vi "Dequeue.vi"(8 "ErrorArray In":errorcluster[](array[cluster])) -> (0 "ErrorArray Out":errorcluster[](array[cluster]), 1 "Data":variant, 2 "Msg":string)   [LabVIEW 2014, in "Bus.lvlib" / "NISTBus.lvclass"]
uses:
  NISTBus.lvclass
  Framework/MsgQueue/TypeDef/MsgQueue.ctl
  <vilib>/Utility/error.llb/Error Cluster From Error Code.vi
  <vilib>/ErrorRing/Error Ring.xnode
  Framework/TestFramework.lvlib
  <userlib>/NIST/NISTErrorLib/NISTErrorLib.lvlib
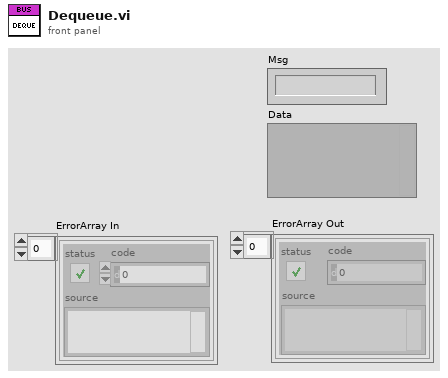
[diagram p1: front panel]
types:
  T1 = typedef "TestFramework.lvlib/MsgQueue.ctl" = cluster{"Msg":string, "Data":variant}
  T2 = typedef "TestFramework.lvlib/QueRef.ctl" = refnum<queue>
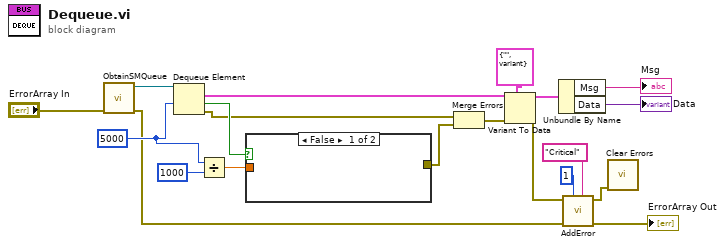
[diagram p0: block diagram]
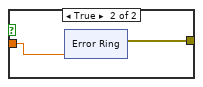
[diagram p2: hidden frame]
diagram:
  w17 = 5000 ("timeout in ms (-1)")
  n1 = call "ObtainSMQueue.vi"("ErrorArray In"="ErrorArray In") -> ("ErrorArray Out"=w4:errorcluster[], "QueRef"=w19:T2)  [unwired: 9 in]
  n2 = Dequeue Element(queue=w19, timeout in ms (-1)=w17) -> (element=w1:T1, timed out?=w16:bool, error out=w13:errorcluster)  [unwired: 1 in, 1 out]
  n3 = Divide(x=w17, y=1000) -> (x/y=w15:dbl)
  n4 = case shown="False" w16 {
    tunnel: w15 -> [_ w22]
    tunnel: [_ w21] -> w14
    frame False {
    }
    frame True {
      n5 = xnode "Error Ring"("parameter 0"=w22) -> ("error out"=w21:errorcluster)
    }
  }
  n6 = Merge Errors(w13, w14) -> (w12:errorcluster)
  n7 = Variant To Data(error in=w12, type=T1 {"Msg"="", "Data"=variant} ("MsgQueue"), Variant=w1) -> (data=w10:T1, error out=w2:errorcluster)
  n8 = Unbundle By Name(w10) -> ("Msg"=→"Msg":string, "Data"=→"Data":variant)
  n9 = call <userlib>:"AddError.vi"("Severity"="Critical", "Priority"=u8 1, "ErrorArray"=w4, "error in (no error)"=w2) -> ("ErrorArray"=→"ErrorArray Out":errorcluster[], "error out"=w5:errorcluster)  [unwired: 6 in]
  n10 = call <vilib>:"Clear Errors.vi"("error in (no error)"=w5) -> ()  [unwired: 5 in, 2 out]
